vi "LoadMulipageImageGUI.vi"() -> ()   [LabVIEW 2011]
uses:
  <vilib>/vision/Image Controls.llb/IMAQ Image.ctl
  Library/tiff/TiffModules/ReadTiffPage_I16_text.vi
panel:
  in  "Stopp":bool
  in  "Load":bool
  out "IMAQ number":i32
  out "error out":errorcluster
  out "Subimage":i32=1
  in  "Path":path
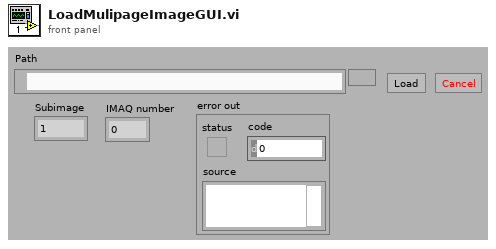
[diagram p1: front panel]
types:
  T1 = typedef "IMAQ Image.ctl" = refnum<image>
  T2 = enum16{"status", "createIMAQ", "getIMAQ", "getNumber", "deleteIMAQ", "deleteAll", "MemoryUsage", "GetAccess", "DecreaseAccess", "ActualIndex"}
  T3 = cluster{"Tiff refnum":refnum<file>, "Byte-Reihenfolge (0:Big-Endian, 2:LSB)":enum16{"big-endian, network order", "native, host order", "little-endian"}}
  T4 = typedef "ScanControl.ctl" = cluster{"Time [s]":dbl, "action":T5, "channel":T6, "value (/s)":dbl}[]
  T5 = typedef "ScanControl_Action.ctl" = enum16{"Abs", "Rel", "Inc", "IncInc", "LoopStart", "LoopEnd", "WaitTriggerRising"}
  T6 = typedef "ScanControl_Channel.ctl" = enum16{"Com", "AnalogConfig", "AnalogValue", "GalvoX", "GalvoY", "Galvo3", "Galvo4", "Digital", "Free", "Loop", "SMoveTime", "Image1X", "Image1Y", "Image2X", "Image2Y"}
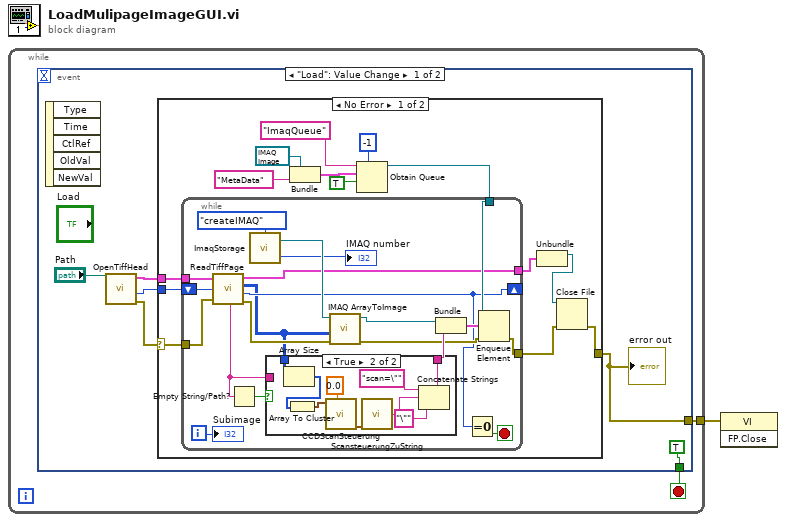
[diagram p0: block diagram]
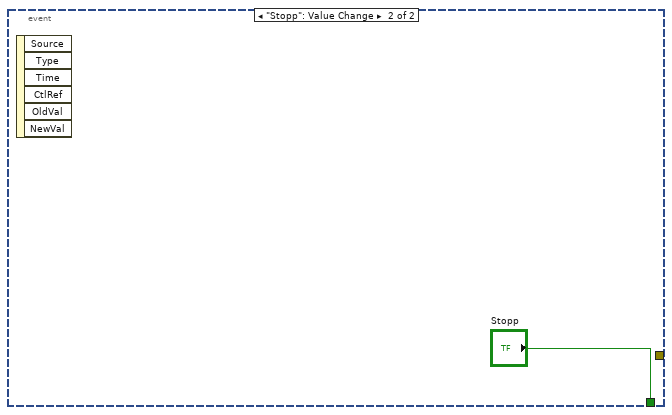
[diagram p4: hidden frame]
diagram:
  n1 = while {
    tunnel: [w2] -> w1
    stop <- w3 stop-if-true
    n2 = event shown="[0] \"Load\": Value Change" {
      selector: _ -> [_ _]
      dyn-events: _ -> [_ _]
      timeout: _ -> [_ _]
      tunnel: [TRUE ("Stopp") "Stopp"] -> w3
      tunnel: [w4 _] -> w2
      event "Load": Value Change {
        n3 = event-data() -> ()  [unwired: 6 out]
        n4 = call "OpenTiffHead.vi"("file path"="Path") -> ("TIFF file"=w7:T3, "first Diroffset"=w5:u32, "error out"=w6:errorcluster)  [unwired: 1 in, 1 out]
        n5 = case shown="No Error" w6 {
          selector: w6 -> [w15 w54]
          tunnel: [w10 w54] -> w4
          tunnel: w7 -> [w16 _]
          tunnel: w5 -> [w14 _]
          frame No Error {
            n6 = Bundle("New Image"=T1 refnum, "MetaData") -> (w19:cluster{"New Image":T1, string})  [unwired: 1 out]
            n7 = Obtain Queue(max queue size (-1, unlimited)=-1, name (unnamed)="ImaqQueue", element data type=w19, create if not found? (T)=TRUE) -> (queue out=w17:refnum<queue>)  [unwired: 1 in, 2 out]
            n8 = while {
              tunnel: w17 -> [w39]
              tunnel: [w36] -> w11
              tunnel: w16 -> [w33]
              tunnel: w15 -> [w26]
              tunnel: [w31] -> w13
              shift-right: [w28] -> _
              shift-left: w14 -> [w30]
              i -> [w29]
              stop <- w27 stop-if-true
              n9 = call-poly "ReadTiffPage.vi"("TIFF file"=w33, "IFDoffset"=w30, "error in"=w26) -> ("TIFF file out"=w31:T3, "16-bit pixmap"=w24:i16[][], "string"=w32:string, "Next offset"=w28:i32, "error out"=w25:errorcluster)  [unwired: 3 out]
              n10 = Empty String/Path?(string/path=w32) -> (empty?=w34:bool)
              n11 = call "ImaqStorage.vi"("Command"=T2."createIMAQ") -> ("Number out"=→"IMAQ number":i32, "IMAQ out"=w41:T1)  [unwired: 2 in]
              n12 = case shown="True" w34 {
                tunnel: [w44 w49] -> w38
                tunnel: w32 -> [w44 _]
                tunnel: w24 -> [_ w45]
                frame False {
                }
                frame True {
                  n13 = Array Size(array=w45) -> (size(s)=w46:i32[])
                  n14 = Array To Cluster(array=w46) -> (cluster=w47:cluster{"[0]":i32, "[1]":i32})
                  n15 = call "CCDScanSteuerung.vi"("Winkel"=0.0, "pixels"=w47) -> ("ScanSteuerung"=w53:T4)  [unwired: 4 in, 5 out]
                  n16 = call "ScansteuerungZuString.vi"("ScanSteuerung neu"=w53) -> ("String"=w51:string)
                  n17 = Concatenate Strings("scan=\"" ("string"), w51, "\"" ("string")) -> (w49:string)
                }
              }
              n18 = call "IMAQ ArrayToImage"("error in (no error)"=w25, "Image Pixels (I16)"=w24, "Image"=w41) -> ("error out"=w37:errorcluster, "Image Out"=w40:T1)  [unwired: 3 in, 4 out]
              n19 = Bundle("Image Out"=w40, "string"=w38) -> (w43:cluster{"Image Out":T1, "string":string})  [unwired: 1 out]
              n20 = Equal To 0?(x=w28) -> (x = 0?=w27:bool)
              n21 = Enqueue Element(queue=w39, element=w43, error in (no error)=w37) -> (error out=w36:errorcluster)  [unwired: 3 out]
              "Subimage" <- w29
            }
            n22 = Unbundle(w13) -> ("Tiff refnum"=w12:refnum<file>)  [unwired: 1 out]
            n23 = Close File(refnum=w12, error in=w11) -> (error out=w10:errorcluster)  [unwired: 1 out]
          }
          frame Error {
          }
        }
        "error out" <- w4
      }
      event "Stopp": Value Change {
        n24 = event-data() -> ()  [unwired: 7 out]
      }
    }
  }
  n25 = invoke class="VI" method="FP.Close"(error in=w1) -> ()  [unwired: 2 in, 3 out]
